vi "XIPIN_Asynchronous_Sample_Rate_Converter_1_0.vi"   [LabVIEW 2017]
doc: "asynchronous sample rate converter (ASRC) converts stereo audio from one sample frequency to another\n------------------------------------\n<b>Need License</b> : No"
uses:
  <vilib>/rvi/XilinxIP/XIPIN_XNode/niFpgaXIPIN.xnode
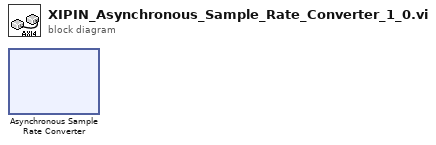
[diagram p0: block diagram]
diagram:
  n1 = xnode ("Asynchronous Sample Rate Converter")() -> ()
